vi "Convert from combo box.vi"(8 "error in (no error)":errorcluster caption="错误输入（无错误）", 10 "CmbBox Ref":refnum<vi>, 11 "Dictionary In":refnum<class "Dictionary.lvclass"> caption="DNL_LabVIEW Object in") -> (0 "error out":errorcluster caption="错误输出", 3 "Dictionary Out":refnum<class "Dictionary.lvclass"> caption="DNL_LabVIEW Object out")   [LabVIEW 2012, in "Dictionary.lvclass"]
uses:
  Dictionary.lvclass
  Dictionary.lvclass/Dictionary.ctl
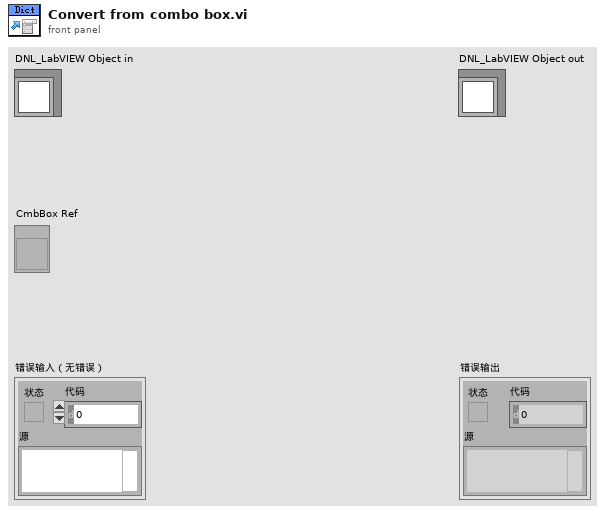
[diagram p1: front panel]
types:
  T1 = typedef "LVComboBoxStrsAndValuesArrayTypeDef.ctl" = cluster{"String":string, "Value":string}[]
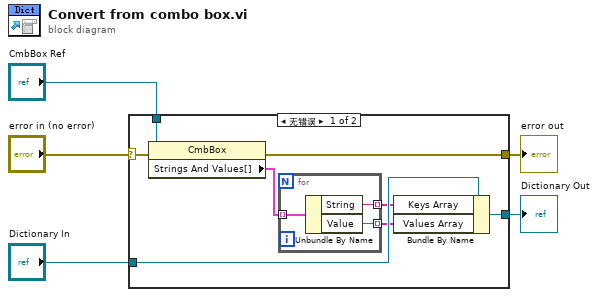
[diagram p0: block diagram]
diagram:
  n1 = case shown="无错误" "error in (no error)" {
    selector: "error in (no error)" -> [w10 w18]
    tunnel: [w9 w18] -> w4
    tunnel: [w12 w17] -> w2
    tunnel: "Dictionary In" -> [w13 w17]
    tunnel: "CmbBox Ref" -> [w11 _]
    frame No Error {
      n2 = property class="CmbBox"(reference=w11, error in=w10) -> (error out=w9:errorcluster, "Strings And Values[]"=w8:T1)  [unwired: 1 out]
      n3 = for {
        tunnel: [w16] -> w7 mode=indexing
        tunnel: [w15] -> w6 mode=indexing
        tunnel: w8 -> [w14] mode=indexing
        n4 = Unbundle By Name(w14) -> ("String"=w16:string, "Value"=w15:string)
      }
      n5 = Bundle By Name(cluster=w13, "Keys Array"=w7, "Values Array"=w6) -> (w12:refnum<class "Dictionary.lvclass">)
    }
    frame Error {
    }
  }
  "error out" <- w4
  "Dictionary Out" <- w2
